vi "StreamEngine.StartCmd.Send.vi"(6 "Project Folder":path, 8 "error in (no error)":errorcluster, 9 "Addon":string, 10 "gRPC ID":T1, 11 "Q Refs":T2) -> (0 "error out":errorcluster)   [LabVIEW 2025, in "XNET Bus Monitor Client.lvlib"]
uses:
  XNET Bus Monitor Client.lvlib
  Types/StreamEngine.CmdQueueData.ctl
  Types/StreamEngine.CmdQueueData.Cmd.ctl
  <vilib>/gRPC/LabVIEW gRPC Library/Shared/grpcId.ctl
  <vilib>/gRPC/LabVIEW gRPC Library/grpc-lvsupport-release.lvlib
  Types/StreamEngine.CmdQueueData.InitialSettings.ctl
  Types/StreamEngine.QueueRefs.ctl
  Types/SubProcessEngine.CmdQueueData.ctl
  Types/SubProcessEngine.CmdQueueData.Cmd.ctl
  Types/SubProcessEngine.QueueRefs.ctl
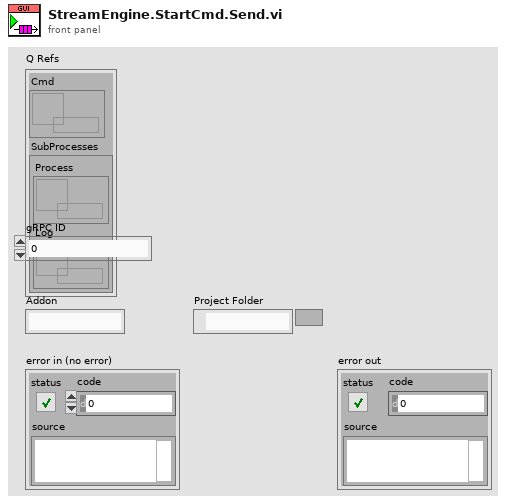
[diagram p1: front panel]
types:
  T1 = typedef "grpc-lvsupport-release.lvlib/grpcId.ctl" = u64
  T2 = typedef "XNET Bus Monitor Client.lvlib/StreamEngine.QueueRefs.ctl" = cluster{"Cmd":refnum<queue>, "SubProcesses":T3}
  T3 = typedef "XNET Bus Monitor Client.lvlib/SubProcessEngine.QueueRefs.ctl" = cluster{"Process":refnum<queue>, "Log":refnum<queue>}
  T4 = typedef "XNET Bus Monitor Client.lvlib/StreamEngine.CmdQueueData.InitialSettings.ctl" = cluster{"gRPC ID":T1, "Addon":string, "Project Folder":path}
  T5 = typedef "XNET Bus Monitor Client.lvlib/StreamEngine.CmdQueueData.Cmd.ctl" = enum8{"Start Stream", "Stop Stream", "Exit"}
  T6 = typedef "XNET Bus Monitor Client.lvlib/StreamEngine.CmdQueueData.ctl" = cluster{"Cmd":T5, "Parameters":variant}
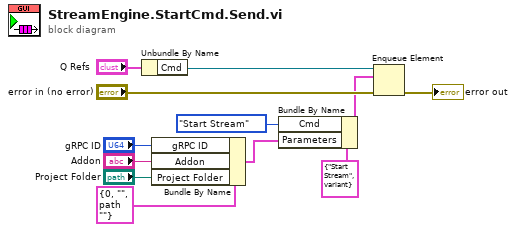
[diagram p0: block diagram]
diagram:
  n1 = Unbundle By Name("Q Refs") -> ("Cmd"=w8:refnum<queue>)
  n2 = Bundle By Name(cluster=T4 {"gRPC ID"=0, "Addon"="", "Project Folder"=path ""}, "gRPC ID"="gRPC ID", "Addon"="Addon", "Project Folder"="Project Folder") -> (w2:T4)
  n3 = Bundle By Name(cluster=T6 {"Cmd"=enum."Start Stream", "Parameters"=variant} ("element"), "Cmd"=StreamEngine.CmdQueueData.Cmd."Start Stream", "Parameters"=w2) -> (w9:T6)
  n4 = Enqueue Element(queue=w8, element=w9, error in (no error)="error in (no error)") -> (error out=→"error out":errorcluster)  [unwired: 1 in, 2 out]
